vi "Your Application.vi"() -> ()   [LabVIEW 2025]
uses:
  Tdef/Product enum.ctl
  SW License Manager.lvlib
  <vilib>/JDP Science/JSONtext/JSONtext.lvlib
  Abstract License/Software License Manager.lvclass
panel:
  in  "stop":bool
  out "License Status":u16(ring)
  out "Note":string
  in  "Controles":dbl
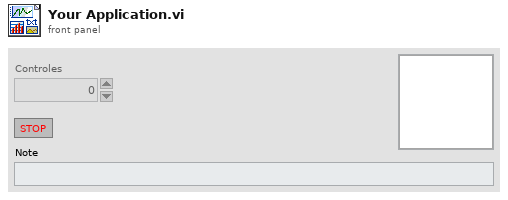
[diagram p1: front panel]
types:
  T1 = typedef "SW License Manager.lvlib/Product enum.ctl" = enum16{"Product_01", "Product_02", "Product_03"}
  T2 = enum8{"Enabled", "Disabled", "Disabled and Grayed Out"}
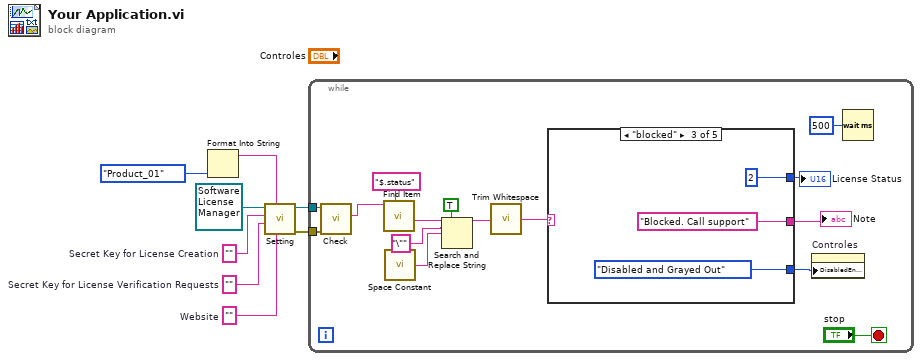
[diagram p0: block diagram]
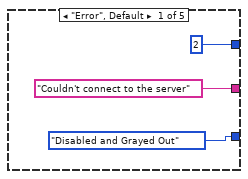
[diagram p2: hidden frame]
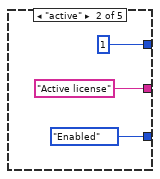
[diagram p3: hidden frame]
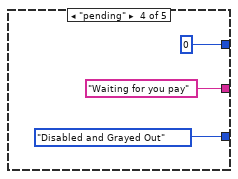
[diagram p4: hidden frame]
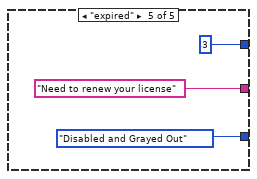
[diagram p5: hidden frame]
diagram:
  w7 = ""  # Secret Key for License Creation
  w6 = ""  # Secret Key for License Verification Requests
  w5 = ""  # Website
  n1 = Format Into String(Product_enum."Product_01" ("Product")) -> (resulting string=w8:string)  [unwired: 3 in, 1 out]
  n2 = call-dynamic "Setting.vi"("Website"=w5, "Product_Ref"=w8, "Secret Key for License Verification Requests"=w6, "Secret Key for License Creation"=w7, "object License in"=refnum<class "Software License Manager.lvclass"> refnum ("Abstract License.lvclass")) -> ("error out"=w4:errorcluster, "Object License out"=w3:refnum<class "Software License Manager.lvclass">)  [unwired: 5 in]
  n3 = while {
    tunnel: w4 -> [w23]
    tunnel: w3 -> [w22]
    stop <- "stop" stop-if-true
    n4 = call-dynamic "Check.vi"("error in (no error)"=w23, "Object License Manager in"=w22) -> ("Body"=w20:string)  [unwired: 6 in, 3 out]
    n5 = call <vilib>:"Find Item.vi"("$Path or Item Name"="$.status", "JSON"=w20) -> ("<JSON>"=w14:string)  [unwired: 6 in, 3 out]
    n6 = call <vilib>:"Space Constant.vi"() -> ("String"=w11:string)
    n7 = Search and Replace String(replace all?=TRUE ("replace all? (F)"), input string=w14, search string="\"", replace string=w11) -> (result string=w10:string)  [unwired: 4 in, 3 out]
    n8 = call <vilib>:"Trim Whitespace.vi"("string"=w10) -> ("trimmed string"=w9:string)  [unwired: 1 in]
    n9 = case shown="\"blocked\"" w9 {
      tunnel: ["Couldn't connect to the server" ("Note") "Active license" ("Note") "Blocked. Call support" ("Note") "Waiting for you pay" ("Note") "Need to renew your license" ("Note")] -> w19
      tunnel: [u16 2 ("License Status") u16 1 ("License Status") u16 2 ("License Status") u16 0 ("License Status") u16 3 ("License Status")] -> w16
      tunnel: [T2."Disabled and Grayed Out" ("DisabledEnum") T2."Enabled" ("DisabledEnum") T2."Disabled and Grayed Out" ("DisabledEnum") T2."Disabled and Grayed Out" ("DisabledEnum") T2."Disabled and Grayed Out" ("DisabledEnum")] -> w15
      frame "Error", Default {
      }
      frame "active" {
      }
      frame "blocked" {
      }
      frame "pending" {
      }
      frame "expired" {
      }
    }
    "Note" <- w19
    "License Status" <- w16
    n10 = property on="Controles" class="DigNum (strict)"("DisabledEnum"=w15) -> ()  [unwired: 2 in, 2 out]
    n11 = Wait (ms)(milliseconds to wait=u32 500) -> ()  [unwired: 1 out]
  }
